vi "getUnregisteredEvents.vi"(8 "error in (no error)":errorcluster, 11 "Event.lvclass in":refnum<class "Event.lvclass">) -> (0 "error out":errorcluster, 2 "unregisteredEvents":string[](array[string]), 3 "Event.lvclass out":refnum<class "Event.lvclass">)   [LabVIEW 2011, in "Events.lvlib" / "Event.lvclass"]
uses:
  Event.lvclass
  Event.lvclass/Event.ctl
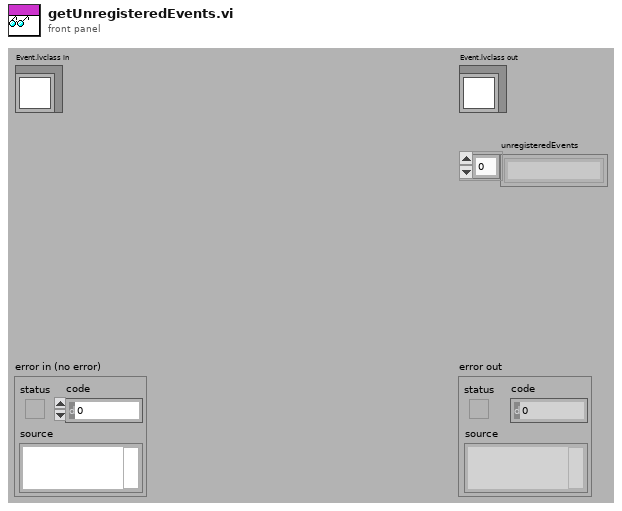
[diagram p1: front panel]
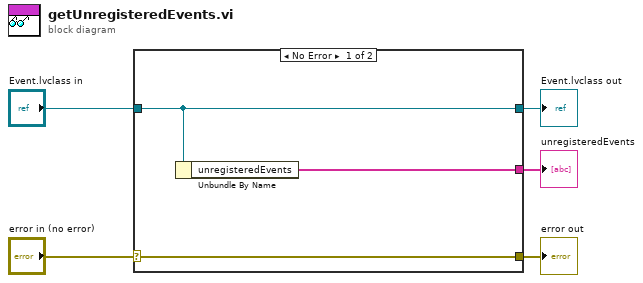
[diagram p0: block diagram]
diagram:
  n1 = case shown="No Error" "error in (no error)" {
    selector: "error in (no error)" -> [w8 w9]
    tunnel: [w8 w9] -> w4
    tunnel: [w7 w10] -> w2
    tunnel: "Event.lvclass in" -> [w7 w10]
    tunnel: [w6 _] -> w1
    frame No Error {
      n2 = Unbundle By Name(w7) -> ("unregisteredEvents"=w6:string[])
    }
    frame Error {
    }
  }
  "error out" <- w4
  "Event.lvclass out" <- w2
  "unregisteredEvents" <- w1
